vi "总磷通讯.vi"() -> ()   [LabVIEW 2016, in "斯坦道总磷.lvlib"]
uses:
  <vilib>/NI/Modbus Library/API/Wrapper/Create TCP Slave.vi
  <vilib>/Utility/config.llb/Write Key (Boolean).vi
  <vilib>/Utility/config.llb/Write Key (String).vi
  <vilib>/Plasmionique/MB Master/MB_Master/MB_Master.lvclass
  <vilib>/NI/Modbus Library/API/slave/Modbus Slave.lvclass
  <vilib>/Utility/config.llb/NI_LVConfig.lvlib
  <vilib>/Plasmionique/MB Master/MB Master.lvlib
  <vilib>/NI/Modbus Library/API/Wrapper/API Main.lvlib
panel:
  out "总氮测量数据区":u16[](array[numeric])
  out "总氮状态告警区":u16[](array[numeric])
  out "总磷状态告警区":u16[](array[numeric])
  out "总磷测量数据区":u16[](array[numeric])
  out "序列号":string
  out "状态告警区":T1 {"告警代码" items=["无告警", "缺试剂告警", "缺水样告警", "缺蒸馏水告警", "缺标液告警", "仪表漏液告警", "标定异常告警", "超量程告警", "加热异常", "低试剂预警", "超上限告警", "超下限告警", "仪表内部其他异常", "滴定异常告警", "电极异常告警", "量程切换告警", "参数设置告警", "PH电极电位异常", "电导率电极异常", "浊度光度异常", "溶解氧电极异常", "溶解氧光强异常", "温度异常告警", "PH异常告警", "溶解氧异常告警", "电导率异常告警", "浊度异常告警", "叶绿素异常告警", "藻密度异常告警", "蓝绿藻异常告警", "ORP异常告警", "氨氮异常告警", "清洁刷异常告警", "SD卡异常告警", "蓝牙异常告警", "Wifi异常告警", "流程异常告警"]; "故障代码" items=["无故障", "电机故障", "温度故障", "通讯故障", "滴定故障"]}
  out "测量数据区":T2 {"单位" items=["ug/L", "mg/L", "ppm", "mg/m3", "cm", "ppb", "ug/m3", "%", "nmol/mol", "umol/mol", "MPN/L", "MPN/100ml", "ng/m3", "NTU", "无量纲", "ms/cm", "us/cm", "℃", "mV", "万个/L"]}
  out "status":bool
  out "关键参数区":T3
  in  "读关键参数区":bool
  in  "读状态告警区":bool
  in  "读测量数据区":bool
  in  "站号":u16(ring) items=["总磷"=1, "氨氮"=3]
  in  "停止":bool
  in  "启动":bool
  in  "控制命令":u16(ring) items=["启动测量"=1, "标样核查"=2, "零点核查"=3, "跨度核查"=4, "空白测试"=5, "平行样测试"=6, "加标回收"=7, "空白校准"=8, "标样校准"=9, "初始化（清洗）"=10, "停止测试"=11, "仪器重启"=12, "校时"=13, "模式设置"=14, "测量间隔设置"=15]
  in  "控制命令参数":u16[](array[numeric]) format="%04xH"
  in  "VISA Resource":refnum<visa-resource-name>
  in  "启用模块":bool
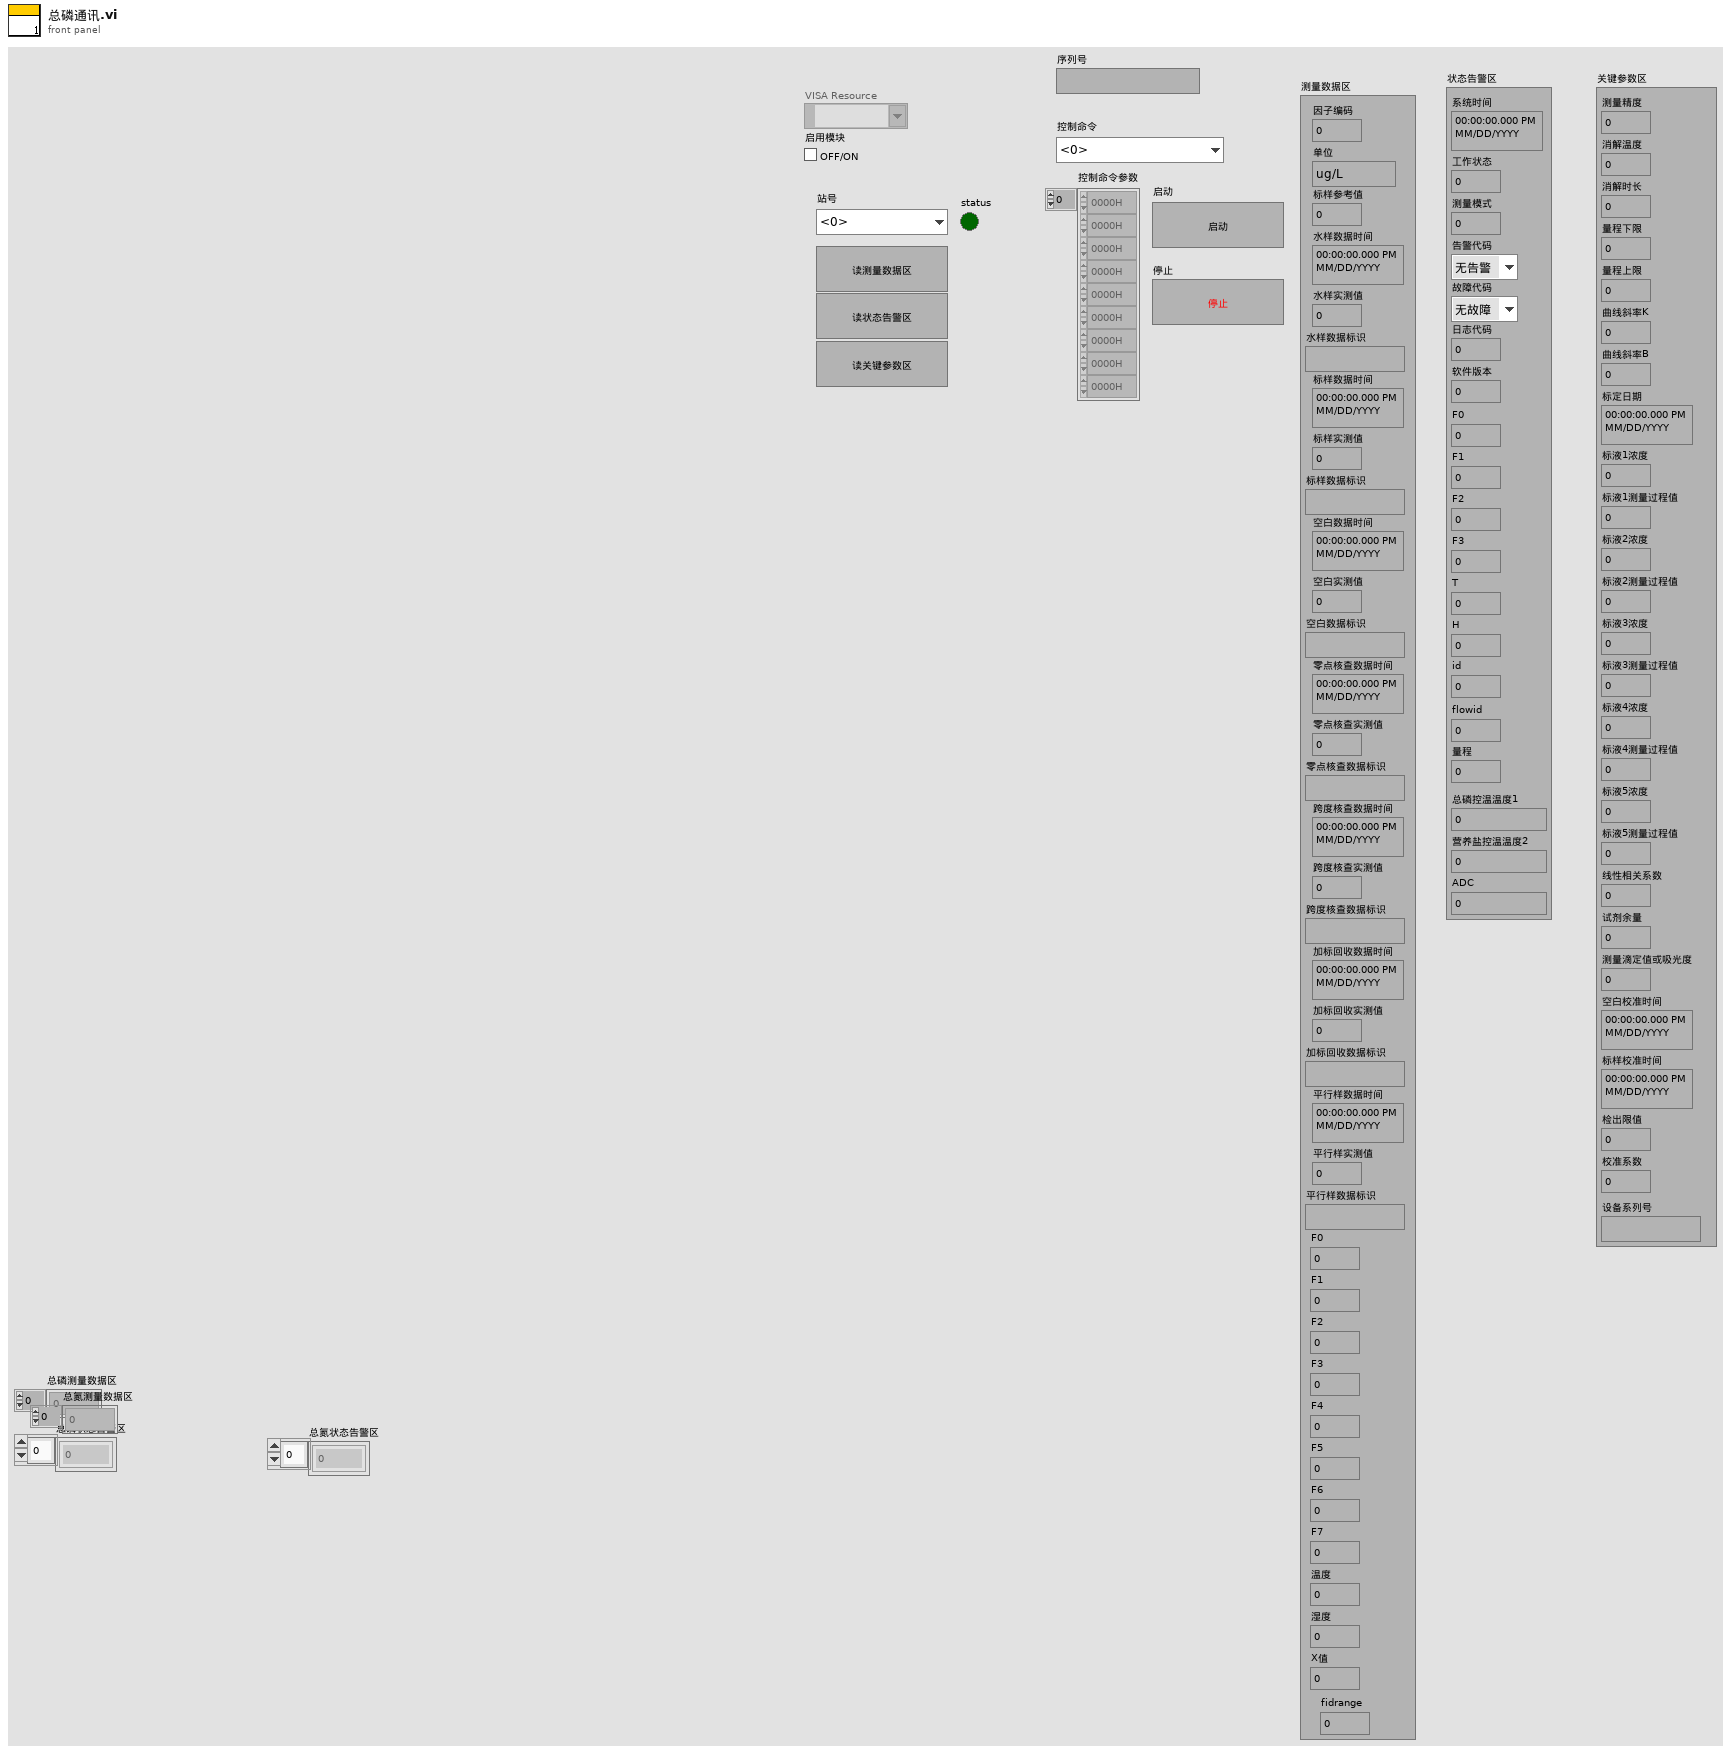
[diagram p1: front panel]
types:
  T1 = cluster{"系统时间":timestamp, "工作状态":u16, "测量模式":u16, "告警代码":u16, "故障代码":u16, "日志代码":u16, "软件版本":u16, "F0":sgl, "F1":sgl, "F2":sgl, "F3":sgl, "T":sgl, "H":sgl, "id":u16, "flowid":u16, "量程":u16, "总磷控温温度1":sgl, "营养盐控温温度2":sgl, "ADC":sgl}
  T2 = cluster{"因子编码":u32, "单位":u16, "标样参考值":sgl, "水样数据时间":timestamp, "水样实测值":sgl, "水样数据标识":string, "标样数据时间":timestamp, "标样实测值":sgl, "标样数据标识":string, "空白数据时间":timestamp, "空白实测值":sgl, "空白数据标识":string, "零点核查数据时间":timestamp, "零点核查实测值":sgl, "零点核查数据标识":string, "跨度核查数据时间":timestamp, "跨度核查实测值":sgl, "跨度核查数据标识":string, "加标回收数据时间":timestamp, "加标回收实测值":sgl, "加标回收数据标识":string, "平行样数据时间":timestamp, "平行样实测值":sgl, "平行样数据标识":string, "F0":sgl, "F1":sgl, "F2":sgl, "F3":sgl, "F4":sgl, "F5":sgl, "F6":sgl, "F7":sgl, "温度":sgl, "湿度":sgl, "X值":sgl, "fidrange":u16}
  T3 = cluster{"测量精度":u16, "消解温度":u16, "消解时长":u16, "量程下限":sgl, "量程上限":sgl, "曲线斜率K":sgl, "曲线斜率B":sgl, "标定日期":timestamp, "标液1浓度":sgl, "标液1测量过程值":sgl, "标液2浓度":sgl, "标液2测量过程值":sgl, "标液3浓度":sgl, "标液3测量过程值":sgl, "标液4浓度":sgl, "标液4测量过程值":sgl, "标液5浓度":sgl, "标液5测量过程值":sgl, "线性相关系数":sgl, "试剂余量":u32, "测量滴定值或吸光度":sgl, "空白校准时间":timestamp, "标样校准时间":timestamp, "检出限值":sgl, "校准系数":sgl, "设备系列号":string}
  T4 = cluster{"水样测试量程模式":enum16{"H", "L", "AUTO"}, "空白核查量程模式":enum16{"H", "L", "AUTO"}, "跨度核查量程模式":enum16{"H", "L", "AUTO"}, "加标回收量程模式":enum16{"H", "L", "AUTO"}}
  T5 = typedef "NI_LVConfig.lvlib/Config Data RefNum.ctl" = refnum<k1>
  T6 = enum8{"Enabled", "Disabled", "Disabled and Grayed Out"}
  T7 = cluster{"系统时间":timestamp, "工作状态":enum16{"空闲", "水样测试", "标样核查", "零点核查", "跨度核查", "空白测试", "平行样测试", "加标回收", "空白校准", "标样校准", "初始化（清洗）"}, "测量模式":enum16{"待机", "连续模式", "周期模式", "定点模式", "受控模式", "手动模式"}, "告警代码":u16, "故障代码":u16, "日志代码":u16, "软件版本":u16, "F0":sgl, "F1":sgl, "F2":sgl, "F3":sgl, "T":sgl, "H":sgl, "id":u16, "flowid":u16, "量程":u16, "总磷控温温度1":sgl, "营养盐控温温度2":sgl, "ADC":sgl}
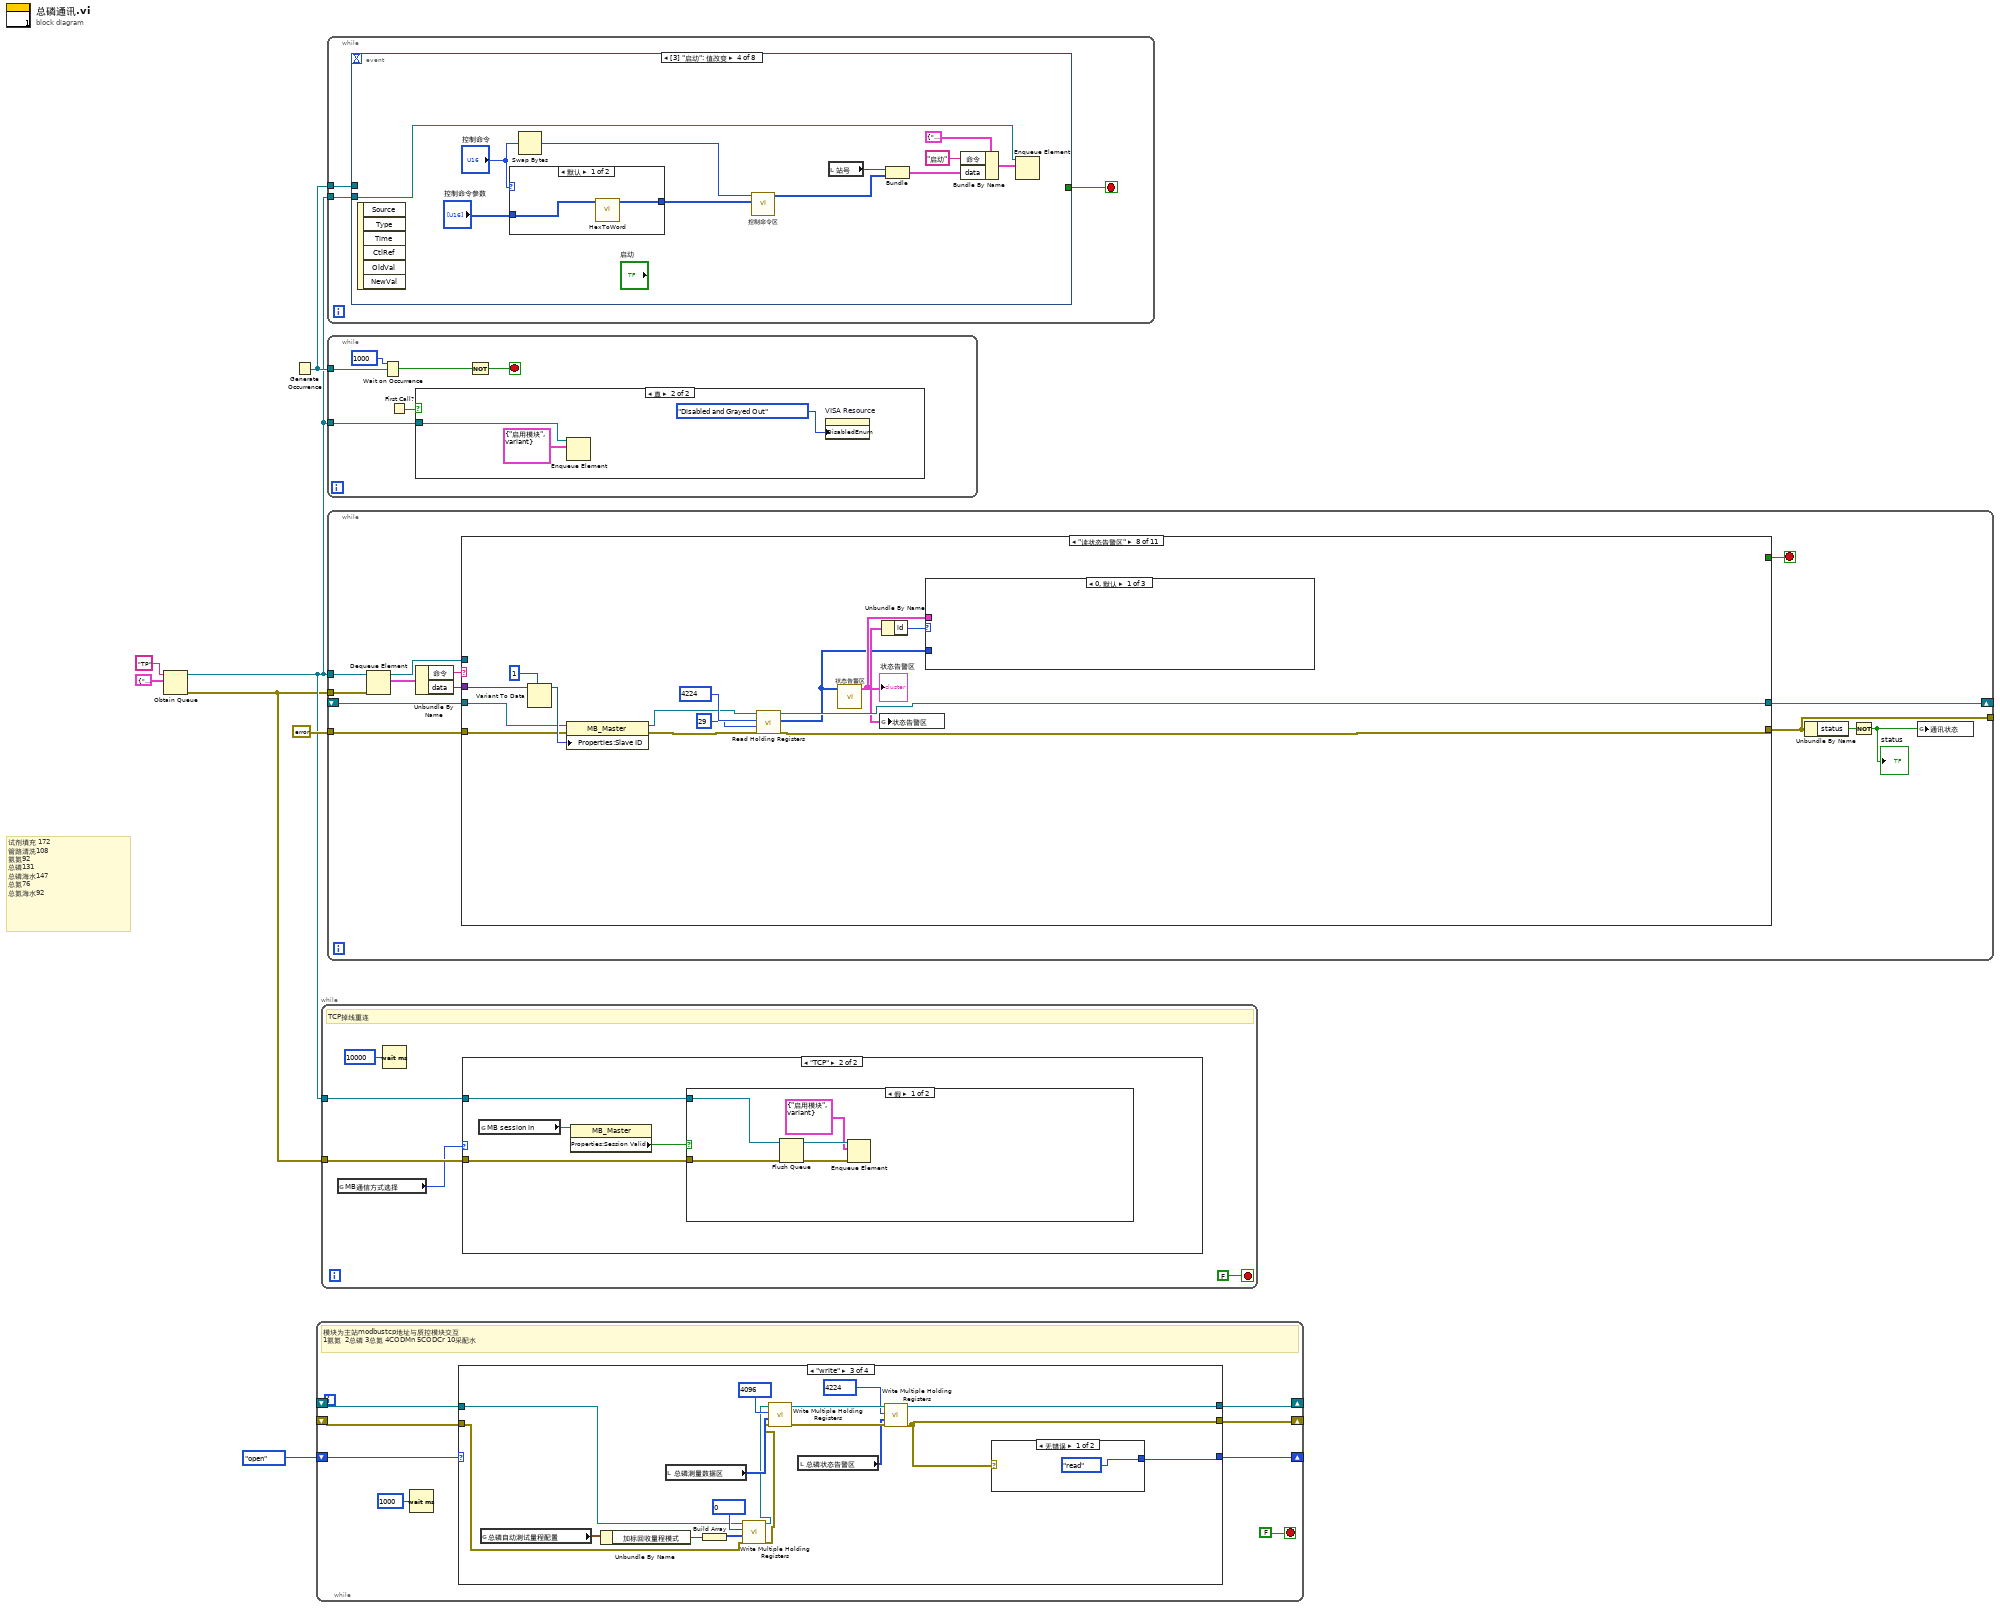
[diagram p0: block diagram]
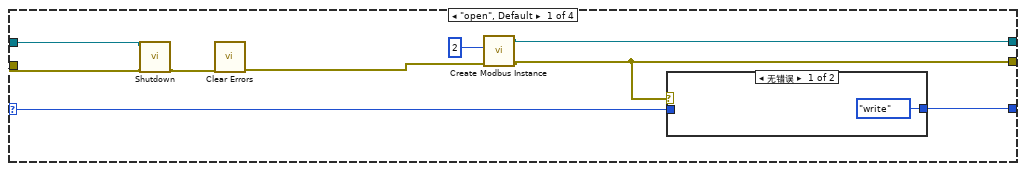
[diagram p4: hidden frame]
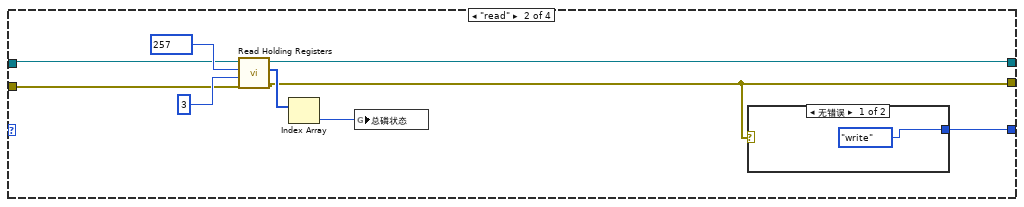
[diagram p6: hidden frame]
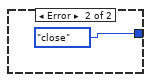
[diagram p7: hidden frame]
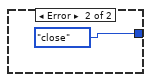
[diagram p8: hidden frame]
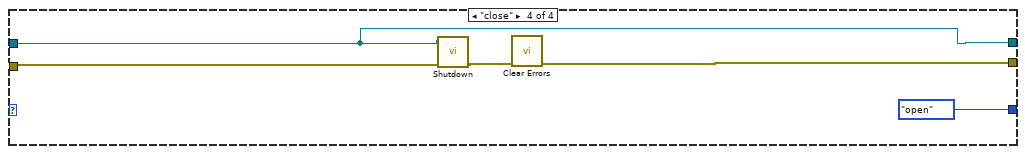
[diagram p9: hidden frame]
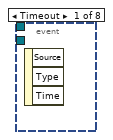
[diagram p11: hidden frame]
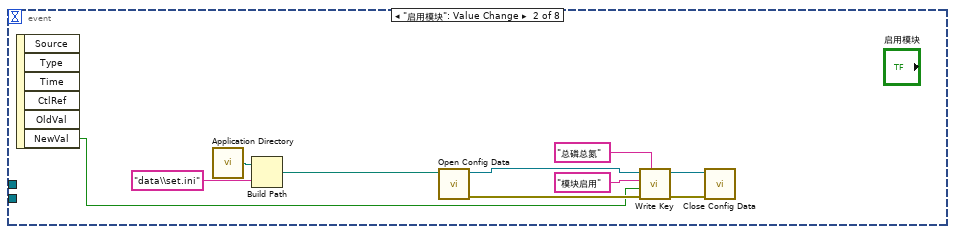
[diagram p12: hidden frame]
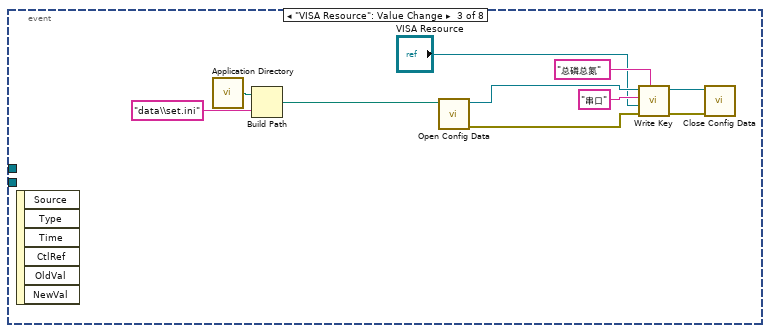
[diagram p13: hidden frame]
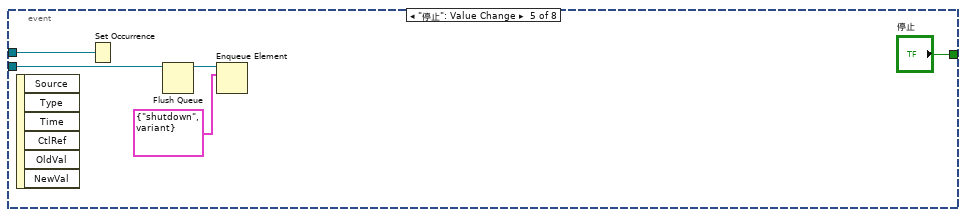
[diagram p15: hidden frame]
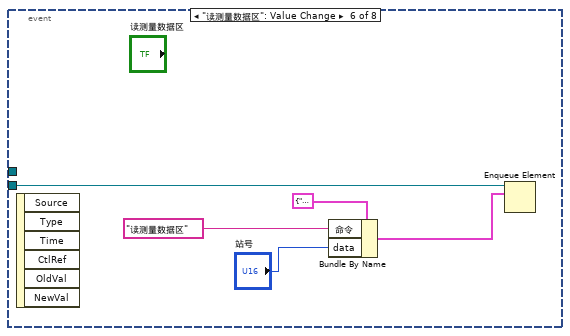
[diagram p16: hidden frame]
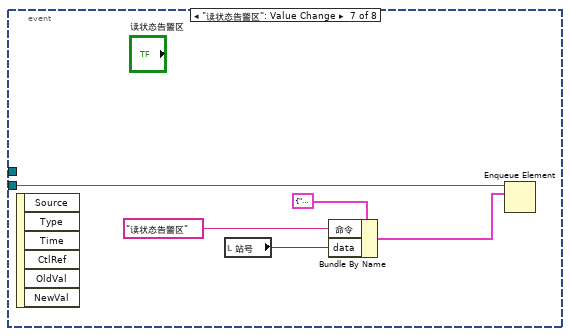
[diagram p17: hidden frame]
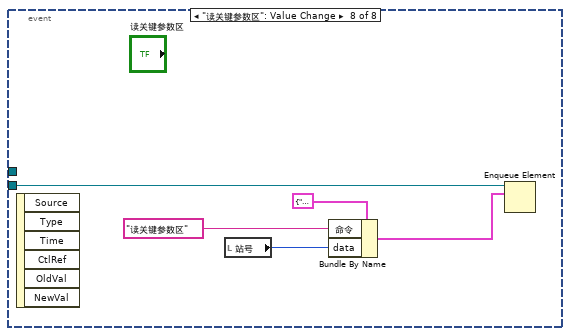
[diagram p18: hidden frame]
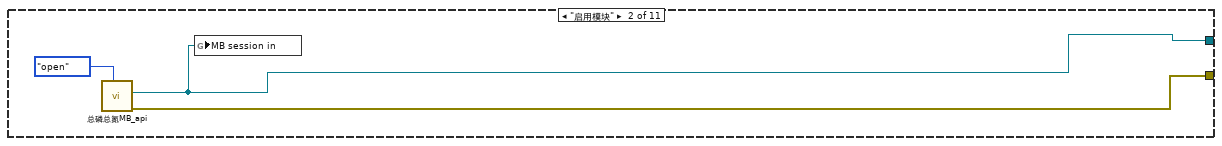
[diagram p20: hidden frame]
diagram:
  # "试剂填充 172 \n管路清洗108\n氨氮92\n总磷131\n总磷海水147\n总氮76\n总氮海水92"
  n1 = Obtain Queue(name (unnamed)="TP" ("名称（未命名）"), element data type=cluster{"命令":string, "data":variant} {"命令"="", "data"=variant}) -> (queue out=w2:refnum<queue>, error out=w1:errorcluster)  [unwired: 3 in, 1 out]
  n2 = Generate Occurrence() -> (w4:refnum<k4>)
  n3 = while {
    shift-right: [w13] -> _
    shift-left: _ -> [w15]
    shift-right: [w12] -> _
    shift-left: _ -> [w14]
    shift-right: [w9] -> _
    shift-left: enum16{"open", "read", "write", "close"}."open" -> [w10]
    stop <- FALSE stop-if-true
    # "模块为主站modbustcp地址与质控模块交互\n1氨氮  2总磷 3总氮 4CODMn 5CODCr 10采配水"
    n4 = Wait (ms)(milliseconds to wait=u32 1000 ("等待时间（毫秒）")) -> ()  [unwired: 1 out]
    n5 = case shown="\"write\"" w10 {
      selector: w10 -> [w24 _ _ _]
      tunnel: w15 -> [w18 w31 w41 w59]
      tunnel: w14 -> [w17 w30 w40 w58]
      tunnel: [w21 w29 w50 w59] -> w13
      tunnel: [w20 w28 w49 w61] -> w12
      tunnel: [w23 w35 w54 enum16{"open", "read", "write", "close"}."open"] -> w9
      frame "open", Default {
        n6 = call-dynamic "Shutdown.vi"("error in"=w17, "Modbus slave in"=w18) -> ("error out"=w16:errorcluster)  [unwired: 9 in]
        n7 = call <vilib>:"Clear Errors.vi"("error in (no error)"=w16) -> ("error out"=w19:errorcluster)  [unwired: 5 in, 1 out]
        n8 = call-poly <vilib>:"Create Modbus Instance.vi"("error in"=w19, "port (502)"=u16 2) -> ("error out"=w20:errorcluster, "TCP slave instance"=w21:refnum<class "Modbus Slave.lvclass">)  [unwired: 8 in]
        n9 = case shown="无错误" w20 {
          tunnel: w24 -> [_ w26]
          tunnel: [enum16{"open", "read", "write", "close"}."write" w26] -> w23
          frame No Error {
          }
          frame Error {
          }
        }
      }
      frame "read" {
        n10 = call-dynamic <vilib>:"Read Holding Registers.vi"("error in"=w30, "number of inputs"=u16 3, "starting address"=u16 257, "Modbus slave in"=w31) -> ("error out"=w28:errorcluster, "register values"=w32:u16[], "Modbus slave out"=w29:refnum<class "Modbus Slave.lvclass">)  [unwired: 5 in]
        n11 = Index Array(array=w32) -> (element=w27:u16)  [unwired: 1 in]
        n12 = global write "VAR总磷全局变量.vi" "总磷状态"(w27) -> ()
        n13 = case shown="无错误" w28 {
          tunnel: [enum16{"open", "read", "write", "close"}."write" enum16{"open", "read", "write", "close"}."close"] -> w35
          frame No Error {
          }
          frame Error {
          }
        }
      }
      frame "write" {
        n14 = global read "总磷断电保存全局变量.vi" "总磷自动测试量程配置"() -> (w43:T4)
        n15 = Unbundle By Name(w43) -> ("加标回收量程模式"=w44:enum16{"H", "L", "AUTO"})
        n16 = local read "总磷测量数据区"() -> (w48:u16[])
        n17 = Build Array(w44) -> (w45:enum16{"H", "L", "AUTO"}[])
        n18 = call-dynamic "Write Multiple Holding Registers.vi"("error in"=w40, "registers to write"=w45, "starting address"=u16 0, "Modbus slave in"=w41) -> ("error out"=w38:errorcluster, "Modbus slave out"=w39:refnum<class "Modbus Slave.lvclass">)  [unwired: 6 in]
        n19 = call-dynamic "Write Multiple Holding Registers.vi"("error in"=w38, "registers to write"=w48, "starting address"=u16 4096, "Modbus slave in"=w39) -> ("error out"=w51:errorcluster, "Modbus slave out"=w52:refnum<class "Modbus Slave.lvclass">)  [unwired: 6 in]
        n20 = local read "总磷状态告警区"() -> (w46:u16[])
        n21 = call-dynamic "Write Multiple Holding Registers.vi"("error in"=w51, "registers to write"=w46, "starting address"=u16 4224, "Modbus slave in"=w52) -> ("error out"=w49:errorcluster, "Modbus slave out"=w50:refnum<class "Modbus Slave.lvclass">)  [unwired: 6 in]
        n22 = case shown="无错误" w49 {
          tunnel: [enum16{"open", "read", "write", "close"}."read" enum16{"open", "read", "write", "close"}."close"] -> w54
          frame No Error {
          }
          frame Error {
          }
        }
      }
      frame "close" {
        n23 = call-dynamic "Shutdown.vi"("error in"=w58, "Modbus slave in"=w59) -> ("error out"=w57:errorcluster)  [unwired: 9 in]
        n24 = call <vilib>:"Clear Errors.vi"("error in (no error)"=w57) -> ("error out"=w61:errorcluster)  [unwired: 5 in, 1 out]
      }
    }
  }
  n25 = while "While循环" {
    tunnel: w2 -> [w64]
    tunnel: w1 -> [w63]
    stop <- FALSE stop-if-true
    # "TCP掉线重连"
    n26 = global read "总磷断电保存全局变量.vi" "MB通信方式选择"() -> (w62:enum16{"串口", "TCP"})
    n27 = Wait (ms)(milliseconds to wait=u32 10000 ("等待时间（毫秒）")) -> ()  [unwired: 1 out]
    n28 = case shown="\"TCP\"" w62 {
      tunnel: w64 -> [_ w69]
      tunnel: w63 -> [_ w68]
      frame "串口", Default {
      }
      frame "TCP" {
        n29 = global read "VAR总磷全局变量.vi" "MB session in"() -> (w67:refnum<class "MB_Master.lvclass">)
        n30 = property class="MB_Master"(reference=w67) -> ("Properties:Session Valid"=w70:bool)  [unwired: 1 in, 2 out]
        n31 = case shown="假" w70 {
          tunnel: w69 -> [w73 _]
          tunnel: w68 -> [w72 _]
          frame False {
            n32 = Flush Queue(queue=w73, error in (no error)=w72) -> (queue out=w75:refnum<queue>, error out=w74:errorcluster)  [unwired: 1 out]
            n33 = Enqueue Element(queue=w75, element=cluster{"命令":string, "data":variant} {"命令"="启用模块", "data"=variant} ("元素"), error in (no error)=w74) -> ()  [unwired: 1 in, 3 out]
          }
          frame True {
          }
        }
      }
    }
  }
  n34 = while {
    tunnel: w2 -> [w78]
    tunnel: w4 -> [w76]
    stop <- w77 stop-if-true
    n35 = event shown="[3] \"启动\": 值改变" {
      selector: _ -> [_ _ _ _ _ _ _ _]
      dyn-events: _ -> [_ _ _ _ _ _ _ _]
      timeout: _ -> [_ _ _ _ _ _ _ _]
      tunnel: w78 -> [_ _ _ w109 w116 w122 w127 w132]
      tunnel: [_ _ _ _ "停止" _ _ _] -> w77
      tunnel: w76 -> [_ _ _ _ w113 _ _ _]
      event Timeout {
        n36 = event-data() -> ()  [unwired: 1 in, 3 out]
      }
      event "启用模块": Value Change {
        n37 = event-data() -> ("NewVal"=w79:bool)  [unwired: 1 in, 5 out]
        n38 = call <vilib>:"Application Directory.vi"() -> ("Application Directory"=w81:path)
        n39 = Build Path(base path=w81, name or relative path="data\\set.ini" ("名称或相对路径")) -> (appended path=w82:path)
        n40 = call <vilib>:"Open Config Data.vi"("configuration file path"=w82) -> ("error out"=w88:errorcluster, "refnum"=w87:T5)  [unwired: 8 in, 1 out]
        n41 = call-poly <vilib>:"Write Key.vi"("section"="总磷总氮", "error in (no error)"=w88, "value"=w79, "key"="模块启用", "refnum"=w87) -> ("error out"=w84:errorcluster, "refnum out"=w80:T5)  [unwired: 4 in, 1 out]
        n42 = call <vilib>:"Close Config Data.vi"("error in (no error)"=w84, "refnum"=w80) -> ()  [unwired: 8 in, 2 out]
      }
      event "VISA Resource": Value Change {
        n43 = event-data() -> ()  [unwired: 1 in, 6 out]
        n44 = call <vilib>:"Application Directory.vi"() -> ("Application Directory"=w91:path)
        n45 = Build Path(base path=w91, name or relative path="data\\set.ini" ("名称或相对路径")) -> (appended path=w92:path)
        n46 = call <vilib>:"Open Config Data.vi"("configuration file path"=w92) -> ("error out"=w98:errorcluster, "refnum"=w97:T5)  [unwired: 8 in, 1 out]
        n47 = call-poly <vilib>:"Write Key.vi"("section"="总磷总氮", "error in (no error)"=w98, "value"="VISA Resource", "key"="串口", "refnum"=w97) -> ("error out"=w94:errorcluster, "refnum out"=w90:T5)  [unwired: 4 in, 1 out]
        n48 = call <vilib>:"Close Config Data.vi"("error in (no error)"=w94, "refnum"=w90) -> ()  [unwired: 8 in, 2 out]
      }
      event "启动": Value Change {
        n49 = event-data() -> ()  [unwired: 1 in, 6 out]
        n50 = case shown="默认" "控制命令" {
          tunnel: "控制命令参数" -> [w111 w112]
          tunnel: [w110 w112] -> w99
          frame Default {
            n51 = call "HexToWord.vi"("数组"=w111) -> ("WORD"=w110:u16[])  [unwired: 10 in]
          }
          frame 13 {
          }
        }
        n52 = Swap Bytes(anything="控制命令") -> (byte swapped=w102:u16)
        n53 = call "控制命令区.vi"("控制命令参数"=w99, "控制命令"=w102) -> ("控制命令"=w105:u16[])  [unwired: 9 in]
        n54 = local read "站号"() -> (w104:u16)
        n55 = Bundle("站号"=w104, "控制命令"=w105) -> (w103:cluster{"站号":u16, "控制命令":u16[]})  [unwired: 1 in]
        n56 = Bundle By Name(cluster=cluster{"命令":string, "data":variant} {"命令"="", "data"=variant} ("元素"), "命令"="启动", "data"=w103) -> (w107:cluster{"命令":string, "data":variant})
        n57 = Enqueue Element(queue=w109, element=w107) -> ()  [unwired: 2 in, 3 out]
      }
      event "停止": Value Change {
        n58 = event-data() -> ()  [unwired: 1 in, 6 out]
        n59 = Set Occurrence(w113) -> ()
        n60 = Flush Queue(queue=w116) -> (queue out=w115:refnum<queue>)  [unwired: 1 in, 2 out]
        n61 = Enqueue Element(queue=w115, element=cluster{"命令":string, "data":variant} {"命令"="shutdown", "data"=variant} ("元素")) -> ()  [unwired: 2 in, 3 out]
      }
      event "读测量数据区": Value Change {
        n62 = event-data() -> ()  [unwired: 1 in, 6 out]
        n63 = Bundle By Name(cluster=cluster{"命令":string, "data":variant} {"命令"="", "data"=variant} ("元素"), "命令"="读测量数据区", "data"="站号") -> (w120:cluster{"命令":string, "data":variant})
        n64 = Enqueue Element(queue=w122, element=w120) -> ()  [unwired: 2 in, 3 out]
      }
      event "读状态告警区": Value Change {
        n65 = event-data() -> ()  [unwired: 1 in, 6 out]
        n66 = local read "站号"() -> (w123:u16)
        n67 = Bundle By Name(cluster=cluster{"命令":string, "data":variant} {"命令"="", "data"=variant} ("元素"), "命令"="读状态告警区", "data"=w123) -> (w125:cluster{"命令":string, "data":variant})
        n68 = Enqueue Element(queue=w127, element=w125) -> ()  [unwired: 2 in, 3 out]
      }
      event "读关键参数区": Value Change {
        n69 = event-data() -> ()  [unwired: 1 in, 6 out]
        n70 = local read "站号"() -> (w128:u16)
        n71 = Bundle By Name(cluster=cluster{"命令":string, "data":variant} {"命令"="", "data"=variant} ("元素"), "命令"="读关键参数区", "data"=w128) -> (w130:cluster{"命令":string, "data":variant})
        n72 = Enqueue Element(queue=w132, element=w130) -> ()  [unwired: 2 in, 3 out]
      }
    }
  }
  n73 = while {
    tunnel: w4 -> [w138]
    tunnel: w2 -> [w134]
    stop <- w135 stop-if-true
    n74 = Wait on Occurrence(2:w138, 3:1000 ("毫秒超时(-1)")) -> (0:w136:bool)  [unwired: 1 in]
    n75 = First Call?() -> (First Call?: T/F=w133:bool)
    n76 = case shown="真" w133 {
      tunnel: w134 -> [_ w140]
      frame False {
      }
      frame True {
        n77 = Enqueue Element(queue=w140, element=cluster{"命令":string, "data":variant} {"命令"="启用模块", "data"=variant} ("元素")) -> ()  [unwired: 2 in, 3 out]
        n78 = property on="VISA Resource" class="VISAName"("DisabledEnum"=T6."Disabled and Grayed Out" ("禁用")) -> ()  [unwired: 2 in, 2 out]
      }
    }
    n79 = Not(x=w136) -> (.not. x?=w135:bool)
  }
  n80 = while {
    tunnel: w2 -> [w154]
    tunnel: w1 -> [w153]
    shift-right: [w151] -> _
    shift-left: _ -> [w150]
    tunnel: errorcluster {"status"=FALSE, "code"=0, "source"=""} ("error out") -> [w149]
    tunnel: [w144] -> _
    stop <- w152 stop-if-true
    n81 = Dequeue Element(queue=w154, error in (no error)=w153) -> (queue out=w145:refnum<queue>, element=w147:cluster{"命令":string, "data":variant})  [unwired: 1 in, 2 out]
    n82 = Unbundle By Name(w147) -> ("命令"=w148:string, "data"=w146:variant)
    n83 = case shown="\"读状态告警区\"" w148 {
      tunnel: w146 -> [_ _ _ w173 w184 w201 w211 w225 w243 w257 _]
      tunnel: w145 -> [_ _ _ _ _ _ _ _ _ _ w270]
      tunnel: [_ _ _ _ _ _ _ _ _ _ TRUE] -> w152
      tunnel: [w155 w158 w160 w176 w187 w203 w215 w234 w250 w264 w266] -> w151
      tunnel: [w156 w157 w161 w175 w186 w202 w216 w224 w251 w265 w267] -> w144
      tunnel: w150 -> [w155 _ w160 w172 w183 w200 w210 w228 w246 w260 w266]
      tunnel: w149 -> [w156 _ w163 w169 w180 w197 w208 w229 w247 w261 w268]
      frame Default {
      }
      frame "启用模块" {
        n84 = call "总磷总氮MB_api.vi"("STEP"=enum16{"open", "read", "write", "close"}."open") -> ("error out"=w157:errorcluster, "MB session out"=w158:refnum<class "MB_Master.lvclass">)  [unwired: 8 in, 1 out]
        n85 = global write "VAR总磷全局变量.vi" "MB session in"(w158) -> ()
      }
      frame "停用模块" {
        n86 = call-dynamic "Close Session.vi"("error in (no error)"=w163, "MB session in"=w160) -> ("error out"=w162:errorcluster)  [unwired: 9 in]
        n87 = call <vilib>:"Clear Errors.vi"("error in (no error)"=w162) -> ("error out"=w161:errorcluster)  [unwired: 5 in, 1 out]
      }
      frame "启动" {
        n88 = Variant To Data(type=cluster{"站号":u16, "控制命令":u16[]} {"站号"=0, "控制命令"=[]} ("输出簇"), Variant=w173) -> (data=w167:cluster{"站号":u16, "控制命令":u16[]})  [unwired: 1 in, 1 out]
        n89 = Unbundle By Name(w167) -> ("站号"=w166:u16, "控制命令"=w164:u16[])
        n90 = property class="MB_Master"(reference=w172, error in=w169, "Properties:Slave ID"=w166) -> (reference out=w171:refnum<class "MB_Master.lvclass">, error out=w170:errorcluster)
        n91 = Index Array(array=w164) -> (element=w165:u16)  [unwired: 1 in]
        n92 = global write "VAR总磷全局变量.vi" "控制命令"(w165) -> ()
        n93 = call <vilib>:"Write Multiple Registers.vi"("error in (no error)"=w170, "values"=w164, "starting address"=u16 4608, "MB session in"=w171) -> ("error out"=w175:errorcluster, "MB session out"=w176:refnum<class "MB_Master.lvclass">)  [unwired: 6 in]
      }
      frame "盲样测试" {
        n94 = Variant To Data(type=0, Variant=w184) -> (data=w177:i32)  [unwired: 1 in, 1 out]
        n95 = case shown="默认" w177 {
          tunnel: [u16[] [] ("values") u16[] [33539, 0] ("values") u16[] [23555, 0] ("values")] -> w179
          frame Default {
          }
          frame 1 {
            # "总磷盲样测试命令"
          }
          frame 3 {
            # "氨氮盲样测试"
          }
        }
        n96 = property class="MB_Master"(reference=w183, error in=w180, "Properties:Slave ID"=w177) -> (reference out=w182:refnum<class "MB_Master.lvclass">, error out=w181:errorcluster)
        n97 = call <vilib>:"Write Multiple Registers.vi"("error in (no error)"=w181, "values"=w179, "starting address"=u16 24592, "MB session in"=w182) -> ("error out"=w186:errorcluster, "MB session out"=w187:refnum<class "MB_Master.lvclass">)  [unwired: 6 in]
      }
      frame "debug" {
        n98 = Variant To Data(type=cluster{"站号":u16, "控制命令":u16[]} {"站号"=0, "控制命令"=[]} ("输出簇"), Variant=w201) -> (data=w195:cluster{"站号":u16, "控制命令":u16[]})  [unwired: 1 in, 1 out]
        n99 = Unbundle By Name(w195) -> ("站号"=w194:u16, "控制命令"=w192:u16[])
        n100 = property class="MB_Master"(reference=w200, error in=w197, "Properties:Slave ID"=w194) -> (reference out=w199:refnum<class "MB_Master.lvclass">, error out=w198:errorcluster)
        n101 = Index Array(array=w192) -> (element=w193:u16)  [unwired: 1 in]
        n102 = global write "VAR总磷全局变量.vi" "控制命令"(w193) -> ()
        n103 = call <vilib>:"Write Multiple Registers.vi"("error in (no error)"=w198, "values"=w192, "starting address"=u16 24594, "MB session in"=w199) -> ("error out"=w202:errorcluster, "MB session out"=w203:refnum<class "MB_Master.lvclass">)  [unwired: 6 in]
      }
      frame "读测量数据区" {
        n104 = Variant To Data(type=u8 1 ("Slave ID"), Variant=w211) -> (data=w206:u8)  [unwired: 1 in, 1 out]
        n105 = property class="MB_Master"(reference=w210, error in=w208, "Properties:Slave ID"=w206) -> (reference out=w209:refnum<class "MB_Master.lvclass">, error out=w207:errorcluster)
        n106 = call <vilib>:"Read Holding Registers.vi"("error in (no error)"=w207, "quantity"=u16 105, "starting address"=u16 4096, "MB session in"=w209) -> ("error out"=w216:errorcluster, "Registers"=w205:u16[], "MB session out"=w215:refnum<class "MB_Master.lvclass">)  [unwired: 5 in]
        n107 = call "测量数据区.vi"("数组"=w205) -> ("测量数据区"=w204:T2)  [unwired: 10 in]
        "测量数据区" <- w204
        n108 = case shown="1" w206 {
          tunnel: w204 -> [_ w217 w219]
          tunnel: w205 -> [_ w218 w220]
          frame 0, Default {
          }
          frame 1 {
            n109 = global write "VAR总磷全局变量.vi" "总磷测量数据区"(w217) -> ()
            "总磷测量数据区" <- w218
          }
          frame 2 {
            n110 = global write "VAR总磷全局变量.vi" "总氮测量数据区"(w219) -> ()
            "总氮测量数据区" <- w220
          }
        }
        n111 = global write "VAR总磷全局变量.vi" "测量数据区"(w204) -> ()
      }
      frame "读状态告警区" {
        n112 = Variant To Data(type=u8 1 ("Slave ID"), Variant=w225) -> (data=w230:u8)  [unwired: 1 in, 1 out]
        n113 = property class="MB_Master"(reference=w228, error in=w229, "Properties:Slave ID"=w230) -> (reference out=w227:refnum<class "MB_Master.lvclass">, error out=w226:errorcluster)
        n114 = call <vilib>:"Read Holding Registers.vi"("error in (no error)"=w226, "quantity"=u16 29, "starting address"=u16 4224, "MB session in"=w227) -> ("error out"=w224:errorcluster, "Registers"=w221:u16[], "MB session out"=w234:refnum<class "MB_Master.lvclass">)  [unwired: 5 in]
        n115 = call "状态告警区.vi"("数组"=w221) -> ("状态告警区"=w222:T7)  [unwired: 10 in]
        "状态告警区" <- w222
        n116 = global write "VAR总磷全局变量.vi" "状态告警区"(w222) -> ()
        n117 = Unbundle By Name(w222) -> ("id"=w223:u16)
        n118 = case shown="0, 默认" w223 {
          tunnel: w222 -> [_ w235 w237]
          tunnel: w221 -> [_ w236 w238]
          frame 0, Default {
          }
          frame 1, 131 {
            n119 = global write "VAR总磷全局变量.vi" "总磷状态告警区"(w235) -> ()
            "总磷状态告警区" <- w236
          }
          frame 2, 76 {
            n120 = global write "VAR总磷全局变量.vi" "总氮状态告警区"(w237) -> ()
            "总氮状态告警区" <- w238
          }
        }
      }
      frame "读关键参数区" {
        n121 = Variant To Data(type=u8 1 ("Slave ID"), Variant=w243) -> (data=w241:u8)  [unwired: 1 in, 1 out]
        n122 = property class="MB_Master"(reference=w246, error in=w247, "Properties:Slave ID"=w241) -> (reference out=w245:refnum<class "MB_Master.lvclass">, error out=w244:errorcluster)
        n123 = call <vilib>:"Read Holding Registers.vi"("error in (no error)"=w244, "quantity"=u16 19, "starting address"=u16 4256, "MB session in"=w245) -> ("error out"=w251:errorcluster, "Registers"=w240:u16[], "MB session out"=w250:refnum<class "MB_Master.lvclass">)  [unwired: 5 in]
        n124 = call "关键参数区.vi"("数组"=w240) -> ("关键参数区"=w239:T3)  [unwired: 10 in]
        "关键参数区" <- w239
        n125 = global write "VAR总磷全局变量.vi" "关键参数区"(w239) -> ()
      }
      frame "读序列号" {
        n126 = Variant To Data(type=u8 1 ("Slave ID"), Variant=w257) -> (data=w255:u8)  [unwired: 1 in, 1 out]
        n127 = property class="MB_Master"(reference=w260, error in=w261, "Properties:Slave ID"=w255) -> (reference out=w259:refnum<class "MB_Master.lvclass">, error out=w258:errorcluster)
        n128 = call <vilib>:"Read Holding Registers.vi"("error in (no error)"=w258, "quantity"=u16 6, "starting address"=u16 4, "MB session in"=w259) -> ("error out"=w265:errorcluster, "Registers"=w254:u16[], "MB session out"=w264:refnum<class "MB_Master.lvclass">)  [unwired: 5 in]
        n129 = call "HexToString.vi"("数组"=w254) -> ("STRING"=w253:string[])  [unwired: 10 in]
        n130 = Index Array(array=w253) -> (element=w252:string)  [unwired: 1 in]
        "序列号" <- w252
        n131 = global write "VAR总磷全局变量.vi" "序列号"(w252) -> ()
      }
      frame "shutdown" {
        n132 = call-dynamic "Close Session.vi"("error in (no error)"=w268, "MB session in"=w266) -> ("error out"=w267:errorcluster)  [unwired: 9 in]
        n133 = Flush Queue(queue=w270) -> (queue out=w269:refnum<queue>)  [unwired: 1 in, 2 out]
        n134 = Release Queue(queue=w269) -> ()  [unwired: 2 in, 3 out]
      }
    }
    n135 = Unbundle By Name(w144) -> ("status"=w143:bool)
    n136 = Not(x=w143) -> (.not. x?=w142:bool)
    "status" <- w142
    n137 = global write "VAR总磷全局变量.vi" "通讯状态"(w142) -> ()
  }
